vi "LBCB Data.vi"(0 "LBCB Number":T1) -> (1 "Cart Data":dbl[](array[numeric]), 2 "Act Data":dbl[](array[numeric]))   [LabVIEW 2009]
uses:
  Data Access Objects/Metadata/LBCB Number.ctl
  Actuator Measurment Actions.ctl
  Cartesian Measurment Actions.ctl
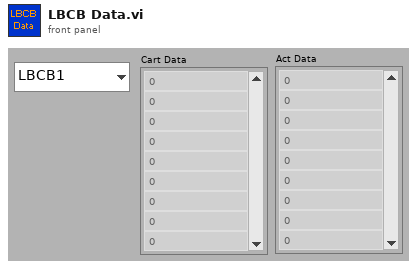
[diagram p1: front panel]
types:
  T1 = typedef "LBCB Number.ctl" = enum16{"LBCB1", "LBCB2"}
  T2 = typedef "Cartesian Measurment Actions.ctl" = enum16{"Set Data", "Get", "Init", "Set Offsets"}
  T3 = typedef "Actuator Measurment Actions.ctl" = enum16{"Set  Data", "Get", "Init"}
  T4 = typedef "Cartesian Data Type.ctl" = cluster{"Displacements":dbl[], "Forces":dbl[], "Displacement Commands":dbl[]}
  T5 = typedef "Actuator DataType.ctl" = cluster{"LVDTs":dbl[], " Commands":dbl[], "Load Cells":dbl[], "Servo":dbl[]}
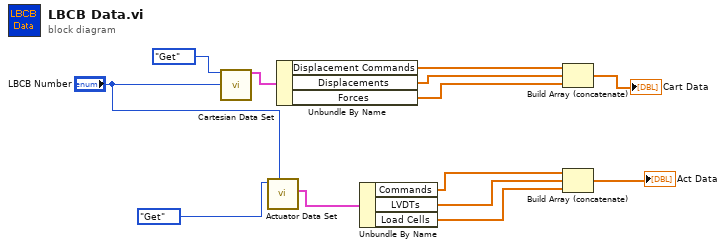
[diagram p0: block diagram]
diagram:
  n1 = call "Cartesian Data Set.vi"("Measurement Actions"=Cartesian_Measurment_Actions."Get", "LBCB Selected"="LBCB Number") -> ("Cartesian Data Out"=w13:T4)  [unwired: 4 in, 9 out]
  n2 = call "Actuator Data Set.vi"("Selected LBCB"="LBCB Number", "Measurement Actions"=Actuator_Measurment_Actions."Get") -> ("Actuator Data Out"=w11:T5)  [unwired: 3 in, 6 out]
  n3 = Unbundle By Name(w13) -> ("Displacement Commands"=w8:dbl[], "Displacements"=w9:dbl[], "Forces"=w10:dbl[])
  n4 = Unbundle By Name(w11) -> ("Commands"=w3:dbl[], "LVDTs"=w2:dbl[], "Load Cells"=w1:dbl[])
  n5 = Build Array (concatenate)(w8, w9, w10) -> (→"Cart Data":dbl[])
  n6 = Build Array (concatenate)(w3, w2, w1) -> (→"Act Data":dbl[])
